vi "Move Menu.vi"(8 "error in (no error)":errorcluster, 10 "Starting Top Position":i32, 11 "MenuButton in":refnum<class "MenuButton.lvclass">) -> (0 "error out":errorcluster, 2 "Ending Bottom Position":i32, 3 "MenuButton out":refnum<class "MenuButton.lvclass">)   [LabVIEW 2017, in "MenuButtons.lvlib" / "MenuButton.lvclass"]
uses:
  MenuButton.lvclass
  MenuButton.lvclass/MenuButton.ctl
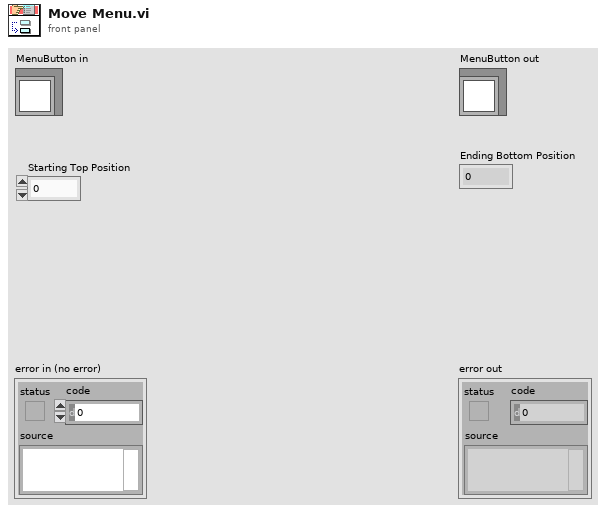
[diagram p1: front panel]
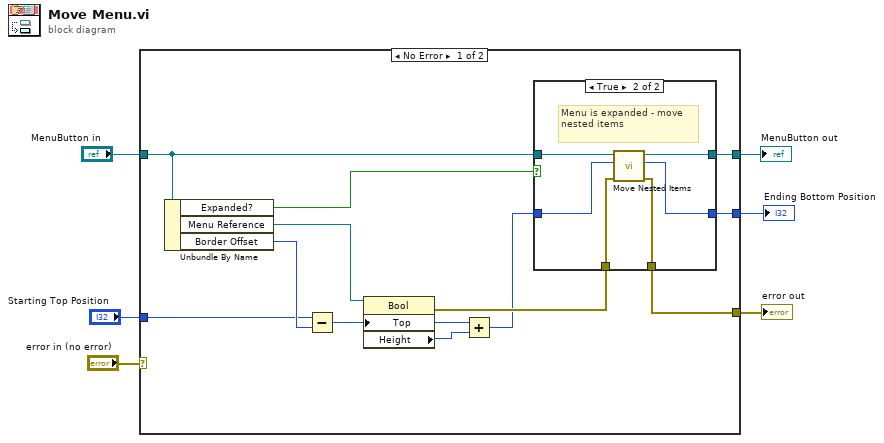
[diagram p0: block diagram]
diagram:
  n1 = case shown="No Error" "error in (no error)" {
    selector: "error in (no error)" -> [_ w28]
    tunnel: [w12 w29] -> w4
    tunnel: "MenuButton in" -> [w18 w29]
    tunnel: "Starting Top Position" -> [w15 _]
    tunnel: [w10 w28] -> w2
    tunnel: [w7 _] -> w1
    frame No Error {
      n2 = Unbundle By Name(w18) -> ("Expanded?"=w9:bool, "Menu Reference"=w17:refnum<vi>, "Border Offset"=w16:i32)
      n3 = Subtract(x=w15, y=w16) -> (x-y=w13:i32)
      n4 = property class="Bool"(reference=w17, "Top"=w13) -> (error out=w11:errorcluster, "Height"=w14:u32)  [unwired: 1 in, 1 out]
      n5 = Add(x=w13, y=w14) -> (x+y=w8:u32)
      n6 = case shown="True" w9 {
        tunnel: w18 -> [w21 w27]
        tunnel: [w21 w26] -> w12
        tunnel: w11 -> [w20 w25]
        tunnel: [w20 w24] -> w10
        tunnel: w8 -> [w19 w23]
        tunnel: [w19 w22] -> w7
        frame False {
          # "Not expanded - dont move nested items"
        }
        frame True {
          # "Menu is expanded - move nested items"
          n7 = call "Move Nested Items.vi"("error in (no error)"=w25, "Starting Top Position"=w23, "MenuButton in"=w27) -> ("error out"=w24:errorcluster, "Ending Bottom Position"=w22:u32, "MenuButton out"=w26:refnum<class "MenuButton.lvclass">)  [unwired: 6 in]
        }
      }
    }
    frame Error {
    }
  }
  "error out" <- w2
  "MenuButton out" <- w4
  "Ending Bottom Position" <- w1
